vi "StringArray2StringList.vi"(1 "String Array":string[](array[string])) -> (0 "String List":string)   [LabVIEW 2019]
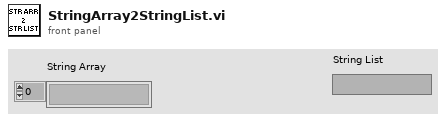
[diagram p1: front panel]
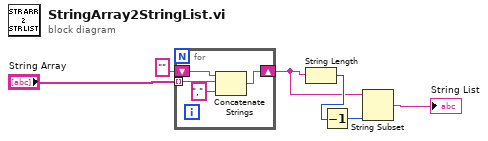
[diagram p0: block diagram]
diagram:
  n1 = for {
    tunnel: "String Array" -> [w10] mode=indexing
    shift-right: [w8] -> w3
    shift-left: "" ("string") -> [w9]
    n2 = Concatenate Strings(w9, w10, "," ("string")) -> (w8:string)
  }
  n3 = String Length(string=w3) -> (length=w4:i32)
  n4 = Decrement(x=w4) -> (x-1=w5:i32)
  n5 = String Subset(string=w3, length (rest)=w5) -> (substring=→"String List":string)  [unwired: 1 in]
